vi "GetIndexNum.vi"(0 "ArrayRef":refnum<vi>, 11 "error in (no error)":errorcluster) -> (4 "ArrayRef out":refnum<vi>, 6 "ItemIndex_row":u32, 8 "ItemIndex_col":u32, 15 "error out":errorcluster)   [LabVIEW 2009]
doc: "To get the index number of the item in a 2D array when you click. \nMake the 2D array have no visible item if posible, because visible items will blink when this VI is called.\nIf the 2D array have no visible item, you can use GetIndexNum_arithemic.vi directly for efficiency.\n\nThis VI is written by Cai Zhibin.\n------------------------------------\nArrayRef: Reference of the 2D array.\nArrayRef out: Pass out the reference.\nItemIndex_row: The Result number (row).\nItemIndex_col: The Result number (column).\nerror in(no error): Error cluster passed in.\nerror out: Pass out the error cluster."
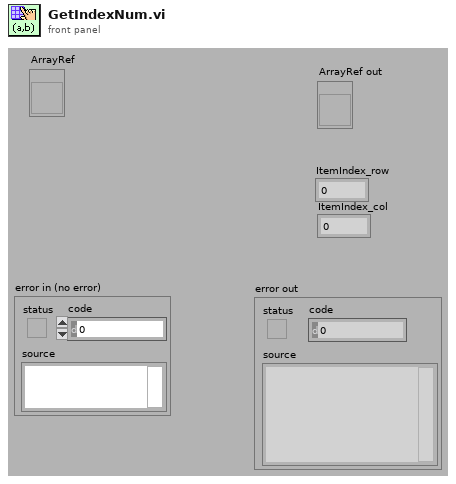
[diagram p1: front panel]
types:
  T1 = typedef "ItemIndex.ctl" = cluster{"Row":i32, "Col":i32}
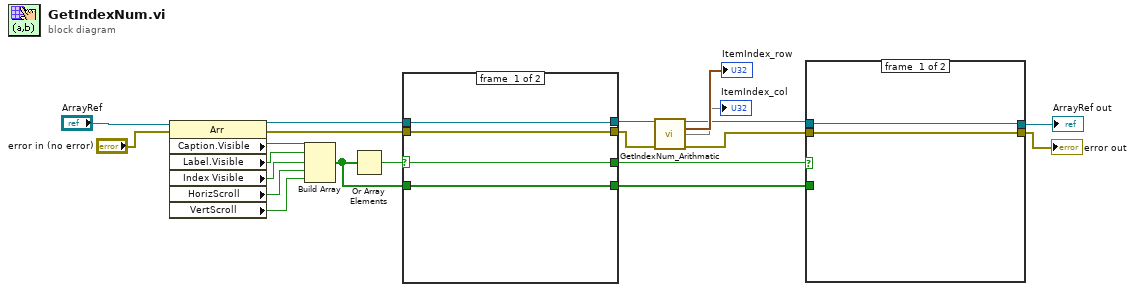
[diagram p0: block diagram]
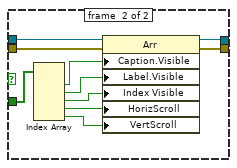
[diagram p2: hidden frame]
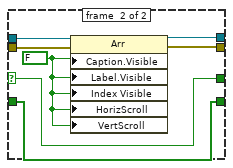
[diagram p3: hidden frame]
diagram:
  n1 = property class="Arr"(reference="ArrayRef", error in="error in (no error)") -> (reference out=w16:refnum<vi>, error out=w15:errorcluster, "Caption.Visible"=w21:bool, "Label.Visible"=w20:bool, "Index Visible"=w19:bool, "HorizScroll"=w18:bool, "VertScroll"=w17:bool)
  n2 = Build Array(w21, w20, w19, w18, w17) -> (w6:bool[])
  n3 = Or Array Elements(Boolean array=w6) -> (logical OR=w10:bool)
  n4 = case shown="True" w10 {
    selector: w10 -> [w23 w27]
    tunnel: w16 -> [w25 w32]
    tunnel: w15 -> [w24 w31]
    tunnel: [w25 w29] -> w2
    tunnel: [w24 w28] -> w11
    tunnel: [w23 w27] -> w7
    tunnel: [w22 w26] -> w5
    tunnel: w6 -> [w22 w26]
    frame #0 {
    }
    frame #1 {
      w30 = FALSE ("Caption.Visible")
      n5 = property class="Arr"(reference=w32, error in=w31, "Caption.Visible"=w30, "Label.Visible"=w30, "Index Visible"=w30, "HorizScroll"=w30, "VertScroll"=w30) -> (reference out=w29:refnum<vi>, error out=w28:errorcluster)
    }
  }
  n6 = call "GetIndexNum_Arithmatic.vi"("ArrayRef"=w2, "error in (no error)"=w11) -> ("ArrayRef out"=w9:refnum<vi>, "ItemIndex"=→"ItemIndex_row":T1, 8:→"ItemIndex_col", "error out"=w8:errorcluster)  [unwired: 10 in]
  n7 = case shown="True" w7 {
    tunnel: w9 -> [w34 w41]
    tunnel: w8 -> [w33 w40]
    tunnel: w5 -> [_ w37]
    tunnel: [w34 w36] -> w1
    tunnel: [w33 w35] -> w4
    frame #0 {
    }
    frame #1 {
      n8 = Index Array(array=w37) -> (element #1=w44:bool, element #2=w42:bool, element #3=w43:bool, element #4=w39:bool, element #5=w38:bool)  [unwired: 5 in]
      n9 = property class="Arr"(reference=w41, error in=w40, "Caption.Visible"=w44, "Label.Visible"=w42, "Index Visible"=w43, "HorizScroll"=w39, "VertScroll"=w38) -> (reference out=w36:refnum<vi>, error out=w35:errorcluster)
    }
  }
  "error out" <- w4
  "ArrayRef out" <- w1
